vi "parseExcel.vi"(0 "module path":path, 1 "function":string, 2 "temp1":string, 3 "temp2":string, 4 "temp3":string, 5 "error in (no error)":errorcluster) -> (14 "return value":string, 19 "error out":errorcluster)   [LabVIEW 2018]
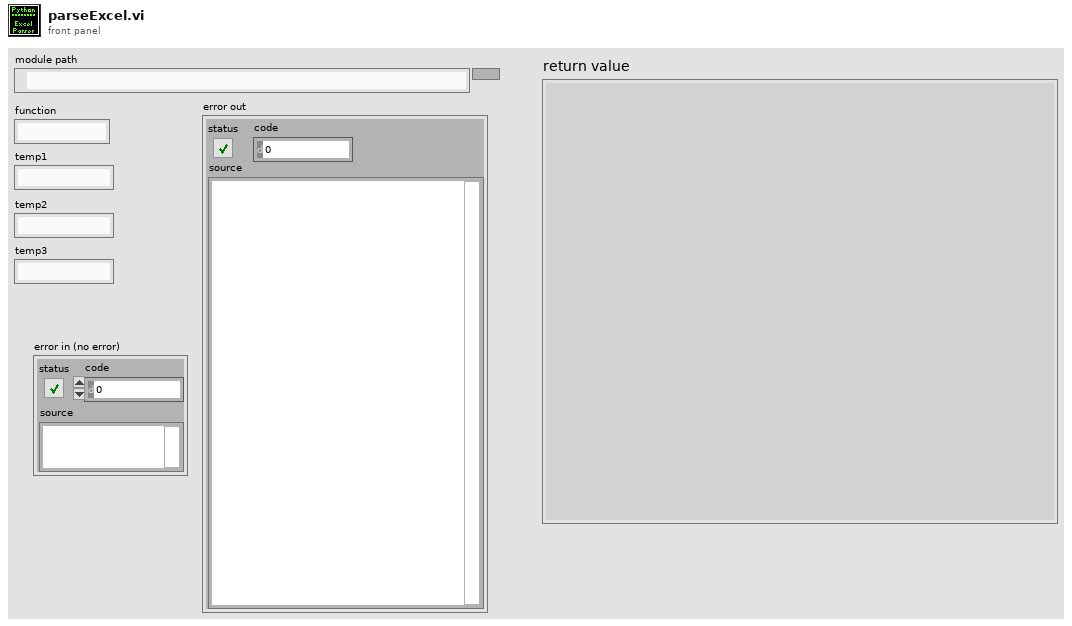
[diagram p1: front panel]
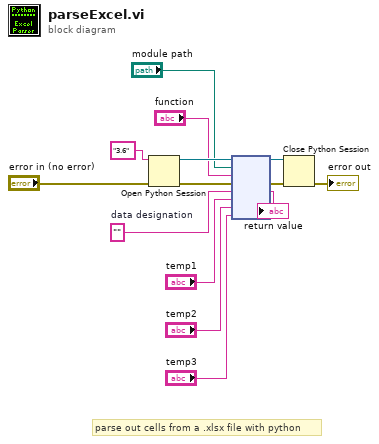
[diagram p0: block diagram]
diagram:
  w10 = ""  # data designation
  # "parse out cells from a .xlsx file with python"
  n1 = Open Python Session(python version="3.6" ("Python version"), 3:"error in (no error)") -> (session out=w14:refnum<k35>, error out=w12:errorcluster)  [unwired: 1 in]
  n2 = node(w14, "module path", "function", w12, w10, "temp1", "temp2", "temp3") -> (w8:refnum<k35>, w7:errorcluster, →"return value":string)  [unwired: 3 in, 2 out]
  n3 = Close Python Session(session in=w8, error in=w7) -> (11:→"error out":errorcluster)
